vi "Big Kahuna.vi"() -> ()   [LabVIEW 2023]
uses:
  9-12-2024/Control 1.ctl
  <vilib>/Utility/file.llb/Write Delimited Spreadsheet (DBL).vi
  <vilib>/Analysis/NI_AALBase.lvlib
panel:
  in  "Reminder":string
  out "Diode st. dev.":dbl format="%0.6f"
  out "Thermistor st. dev.":dbl format="%0.6f"
  out "Diode Mean":dbl format="%0.6f"
  out "Thermistor Mean":dbl format="%0.6f"
  out "Thermocouple st. dev.":dbl format="%0.6f"
  out "Thermocouple Mean":dbl format="%0.6f"
  in  "file path (dialog if empty)":T1
  out "Waveform Chart":cluster{"mean":dbl, "mean":dbl, "mean":dbl}(graph)
  in  "stop (F)":bool
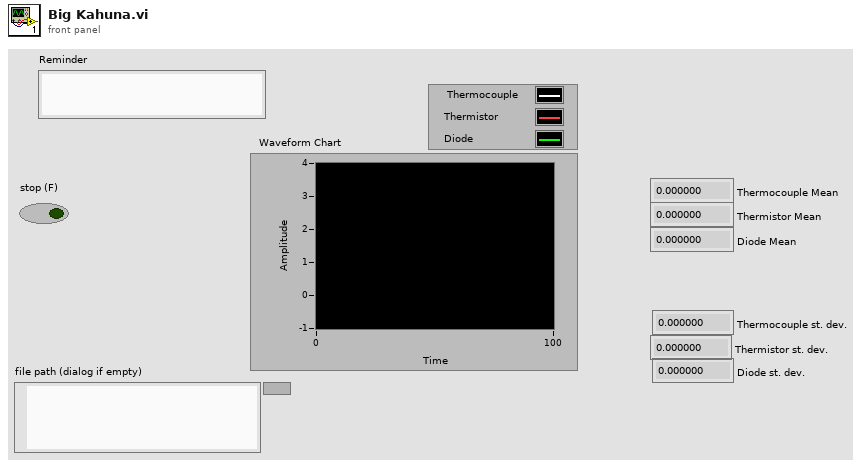
[diagram p1: front panel]
types:
  T1 = typedef "Control 1.ctl" = path
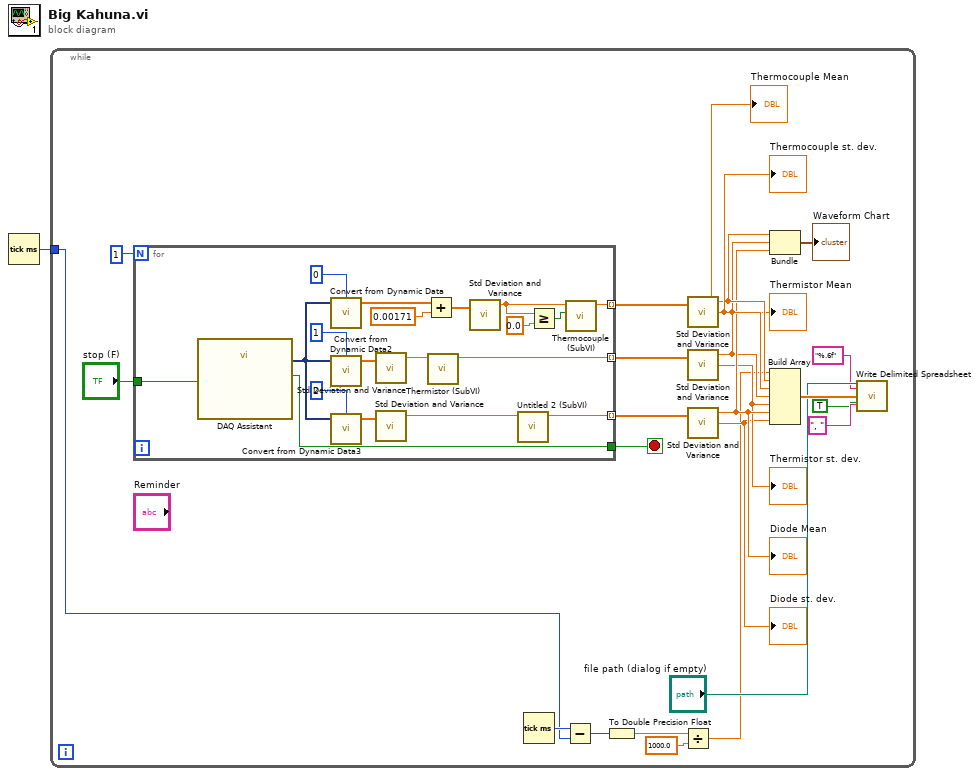
[diagram p0: block diagram]
diagram:
  n1 = Tick Count (ms)() -> (millisecond timer value=w1:u32)
  n2 = while {
    tunnel: w1 -> [w6]
    stop <- w25 stop-if-true
    n3 = for {
      N: 1 -> [_]
      tunnel: [w44] -> w25
      tunnel: [w28] -> w18 mode=indexing
      tunnel: "stop (F)" -> [w37]
      tunnel: [w27] -> w15 mode=indexing
      tunnel: [w26] -> w14 mode=indexing
      n4 = call "DAQ Assistant"("stop (F)"=w37) -> ("data"=w33:dynamicdata, "stopped"=w44:bool)  [unwired: 15 in, 2 out]
      n5 = call "Convert from Dynamic Data"("Dynamic Data Type"=w33, "Channel"=0) -> ("Array"=w40:dbl[])  [unwired: 2 in]
      n6 = call "Convert from Dynamic Data2"("Dynamic Data Type"=w33, "Channel"=1) -> ("Array"=w32:dbl[])  [unwired: 2 in]
      n7 = call "Convert from Dynamic Data3"("Dynamic Data Type"=w33, "Channel"=2) -> ("Array"=w29:dbl[])  [unwired: 2 in]
      n8 = call <vilib>:"Std Deviation and Variance.vi"("X"=w32) -> ("mean"=w31:dbl)  [unwired: 1 in, 2 out]
      n9 = call <vilib>:"Std Deviation and Variance.vi"("X"=w29) -> ("mean"=w30:dbl)  [unwired: 1 in, 2 out]
      n10 = Add(x=w40, y=0.00171) -> (x+y=w41:dbl[])
      n11 = call "Thermistor (SubVI).vi"("mean"=w31) -> ("T"=w27:dbl)  [unwired: 10 in]
      n12 = call <vilib>:"Std Deviation and Variance.vi"("X"=w41) -> ("mean"=w39:dbl)  [unwired: 1 in, 2 out]
      n13 = call "Untitled 2 (SubVI).vi"("mean"=w30) -> ("T"=w26:dbl)  [unwired: 10 in]
      n14 = Greater Or Equal?(x=w39, y=0.0) -> (x >= y?=w38:bool)
      n15 = call "Thermocouple (SubVI).vi"("Boolean"=w38, "mean"=w39) -> ("T"=w28:dbl)  [unwired: 9 in]
    }
    n16 = Tick Count (ms)() -> (millisecond timer value=w7:u32)
    n17 = Subtract(x=w7, y=w6) -> (x-y=w5:u32)
    n18 = To Double Precision Float(number=w5) -> (double precision float=w4:dbl)
    n19 = Divide(x=w4, y=1000.0) -> (x/y=w3:dbl)
    n20 = call <vilib>:"Std Deviation and Variance.vi"("X"=w18) -> ("mean"=w13:dbl, "standard deviation"=w17:dbl)  [unwired: 1 in, 1 out]
    "Thermocouple Mean" <- w13
    "Thermocouple st. dev." <- w17
    n21 = call <vilib>:"Std Deviation and Variance.vi"("X"=w15) -> ("mean"=w10:dbl, "standard deviation"=w9:dbl)  [unwired: 1 in, 1 out]
    "Thermistor Mean" <- w10
    "Thermistor st. dev." <- w9
    n22 = call <vilib>:"Std Deviation and Variance.vi"("X"=w14) -> ("mean"=w11:dbl, "standard deviation"=w8:dbl)  [unwired: 1 in, 1 out]
    "Diode Mean" <- w11
    "Diode st. dev." <- w8
    n23 = Bundle("mean"=w13, "mean"=w10, "mean"=w11) -> (→"Waveform Chart":cluster{"mean":dbl, "mean":dbl, "mean":dbl})  [unwired: 1 in]
    n24 = Build Array(w3, w13, w17, w10, w9, w11, w8) -> (w24:dbl[])
    n25 = call-poly <vilib>:"Write Delimited Spreadsheet.vi"("file path (dialog if empty)"="file path (dialog if empty)", "format (%.3f)"="%.6f", "1D data"=w24, "append to file? (new file:F)"=TRUE, "delimiter (\\t)"=", " ("delimiter (\\t)")) -> ()  [unwired: 9 in, 2 out]
  }
